vi "RTS Populate Cool Dehum Temps Standard Test.vi"(8 "Error In":errorcluster, 11 "Current Test Input":T1 {"Chamber 1-1"."Start Time" format="%<%X\n%x>T"; "Chamber 1-1"."End Time" format="%<%X\n%x>T"; "Chamber 1-2"."Start Time" format="%<%X\n%x>T"; "Chamber 1-2"."End Time" format="%<%X\n%x>T"; "Chamber 1-3"."Start Time" format="%<%X\n%x>T"; "Chamber 1-3"."End Time" format="%<%X\n%x>T"}) -> (0 "Error Out":errorcluster, 3 "Current Test Output":T1 {"Chamber 1-1"."Start Time" format="%<%X\n%x>T"; "Chamber 1-1"."End Time" format="%<%X\n%x>T"; "Chamber 1-2"."Start Time" format="%<%X\n%x>T"; "Chamber 1-2"."End Time" format="%<%X\n%x>T"; "Chamber 1-3"."Start Time" format="%<%X\n%x>T"; "Chamber 1-3"."End Time" format="%<%X\n%x>T"})   [LabVIEW 2020]
uses:
  Type Definitions/RTS Door Op Data.ctl
  Type Definitions/RTS Door Ops Client.ctl
  Type Definitions/RTS Door Opening Schedule.ctl
  Type Definitions/RTS Door Ops Sequence.ctl
  Type Definitions/RTS Standard Door Opening Test.ctl
panel:
  # "Chamber Conditions:"
  # "Chamber Conditions:"
  # "Chamber Conditions:"
  # "Chamber Conditions:"
  # "Chamber Conditions:"
  # "Chamber Conditions:"
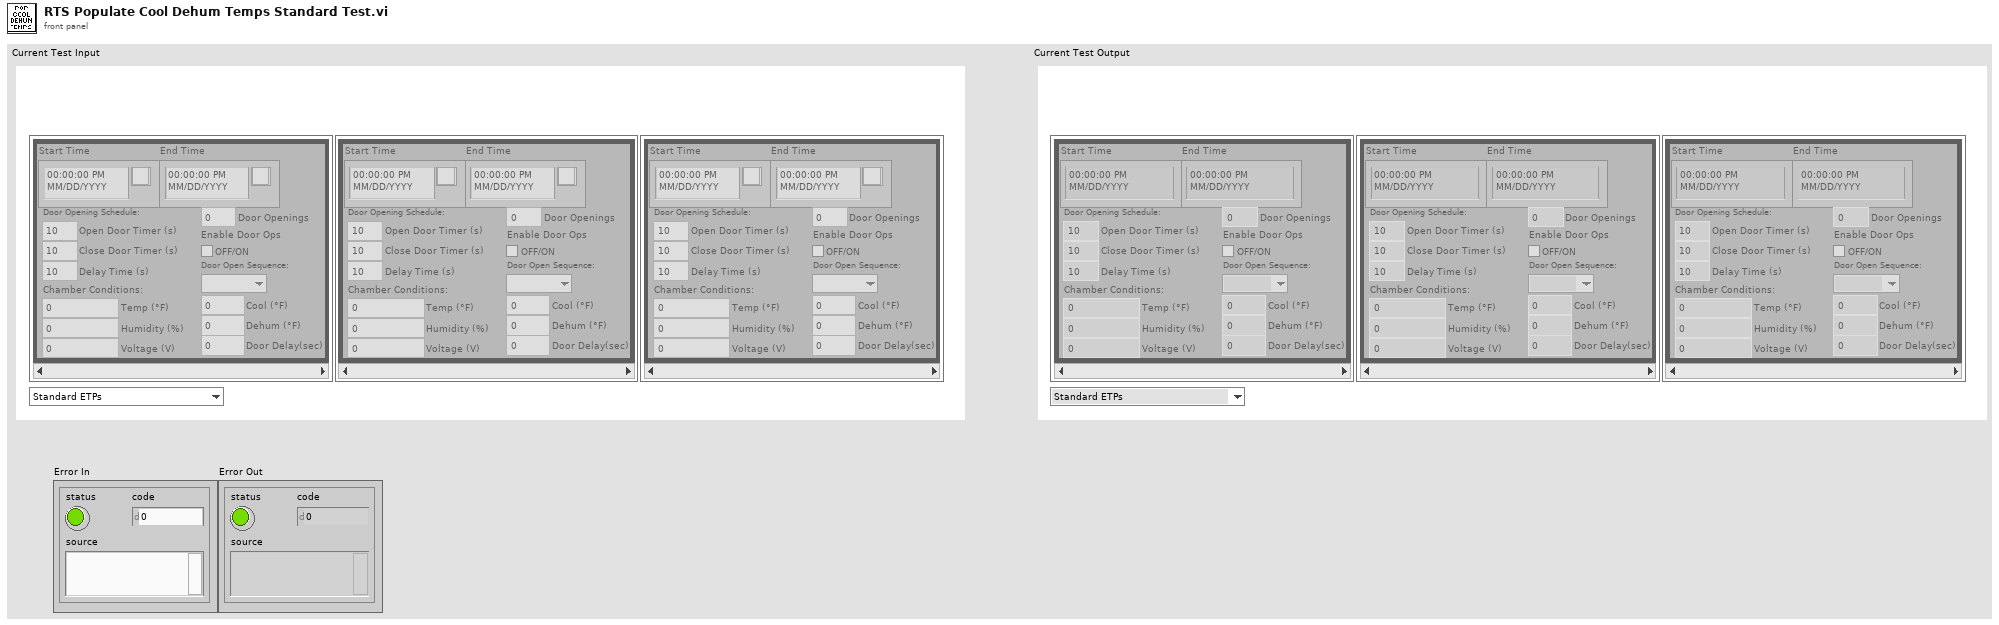
[diagram p1: front panel]
types:
  T1 = typedef "RTS Door Op Data.ctl" = cluster{"Chamber 1-3":T2[], "Chamber 1-2":T2[], "Chamber 1-1":T2[], "Standard Tests 1-1":T5}
  T2 = typedef "RTS Door Ops Client.ctl" = cluster{"End Time":timestamp, "Start Time":timestamp, "Door Opening Schedule:":T3, "Enable Door Ops":bool, "Door Openings":u32, "Temp (°F)":dbl, "Humidity (%)":dbl, "Voltage (V)":dbl, "Door Open Sequence:":T4, "Door Delay(sec)":dbl, "Dehum (°F)":dbl, "Cool (°F)":dbl}
  T3 = typedef "RTS Door Opening Schedule.ctl" = cluster{"Open Door Timer (s)":dbl, "Delay Time (s)":dbl, "Close Door Timer (s)":dbl}
  T4 = typedef "RTS Door Ops Sequence.ctl" = enum16{"", "1st", "2nd", "3rd"}
  T5 = typedef "RTS Standard Door Opening Test.ctl" = enum16{"Standard ETPs", "511-B113 EHUT", "511-B110 HUT", "512-C410 SLAT", "511-B111 Internal Moisture", "511-C401 Moisture Accumulation", "511-B100 No Door Opening (NDO)", "511-B304 ISO Energy Consumption", "Custom Test", "Cancel Test"}
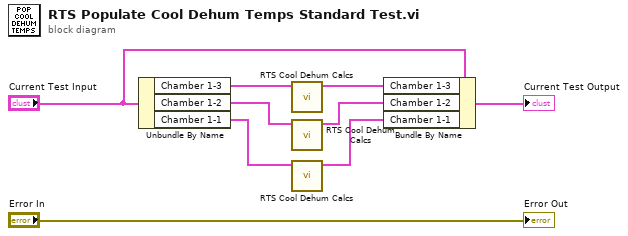
[diagram p0: block diagram]
diagram:
  n1 = Unbundle By Name("Current Test Input") -> ("Chamber 1-3"=w8:T2[], "Chamber 1-2"=w5:T2[], "Chamber 1-1"=w4:T2[])
  n2 = call "RTS Cool Dehum Calcs.vi"("Chamber 1-3"=w8) -> ("Array"=w6:T2[])  [unwired: 10 in]
  n3 = call "RTS Cool Dehum Calcs.vi"("Chamber 1-3"=w5) -> ("Array"=w3:T2[])  [unwired: 10 in]
  n4 = call "RTS Cool Dehum Calcs.vi"("Chamber 1-3"=w4) -> ("Array"=w2:T2[])  [unwired: 10 in]
  n5 = Bundle By Name(cluster="Current Test Input", "Chamber 1-3"=w6, "Chamber 1-2"=w3, "Chamber 1-1"=w2) -> (→"Current Test Output":T1)
  "Error Out" <- "Error In"
